vi "Clear Markers.vi"(0 "VISA Resource Name":refnum<visa-resource-name>, 1 "File Name (WAVEFORM_SEQ)":string="WAVEFORM_SEQ", 2 "Mark Number (1)":u16=1, 3 "First Point (1)":i32=1, 4 "Last Point (1)":i32=1, 5 "error in (no error)":errorcluster {"code" format="%.0x"}, 6 "Clear Type (0: All)":enum16{"All", "Partial"}(ring)) -> (14 "VISA Resource Name Out":refnum<visa-resource-name>, 19 "error out":errorcluster {"code" format="%.0x"})   [LabVIEW 2014, in "Agilent ESG Series.lvlib"]
doc: "This VI clear markers from a waveform segment.\n\nNotes:\n(1) This VI is valid only on instruments Agilent E44xB with the UND option or on instrument E4438C with option 001/601 or 002/602."
uses:
  Agilent ESG Series.lvlib
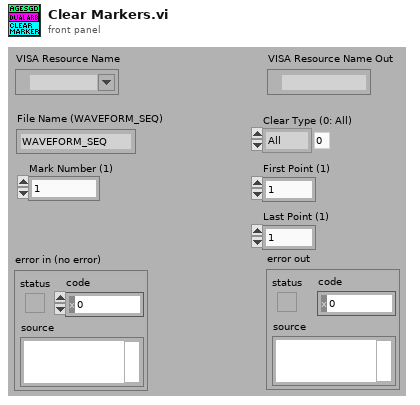
[diagram p1: front panel]
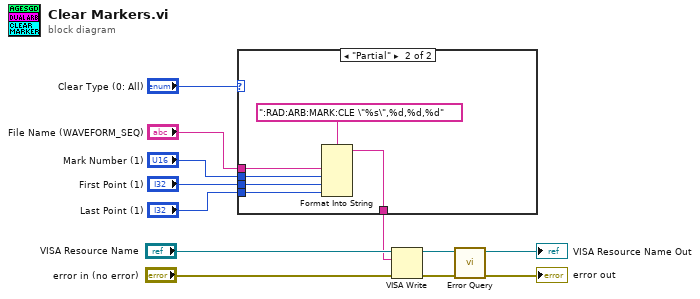
[diagram p0: block diagram]
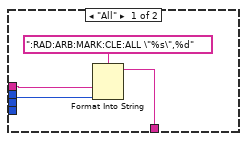
[diagram p2: hidden frame]
diagram:
  n1 = case shown="\"Partial\"" "Clear Type (0: All)" {
    tunnel: "File Name (WAVEFORM_SEQ)" -> [w15 w21]
    tunnel: "Mark Number (1)" -> [w14 w20]
    tunnel: "First Point (1)" -> [_ w19]
    tunnel: "Last Point (1)" -> [_ w18]
    tunnel: [w13 w17] -> w5
    frame "All" {
      n2 = Format Into String(format string=":RAD:ARB:MARK:CLE:ALL \"%s\",%d", w15, w14) -> (resulting string=w13:string)  [unwired: 2 in, 1 out]
    }
    frame "Partial" {
      n3 = Format Into String(format string=":RAD:ARB:MARK:CLE \"%s\",%d,%d,%d", w21, w20, w19, w18) -> (resulting string=w17:string)  [unwired: 2 in, 1 out]
    }
  }
  n4 = VISA Write(VISA resource name="VISA Resource Name", write buffer=w5, error in (no error)="error in (no error)") -> (VISA resource name out=w3:refnum<visa-resource-name>, error out=w4:errorcluster)  [unwired: 1 out]
  n5 = call "Error Query.vi"("VISA Resource Name"=w3, "error in (no error)"=w4) -> ("VISA Resource Name Out"=→"VISA Resource Name Out":refnum<visa-resource-name>, "error out"=→"error out":errorcluster)  [unwired: 10 in, 2 out]
